vi "Measurement.vi"(8 "error in (no error)":errorcluster, 9 "Grandeza":string, 10 "Multiplicador":dbl, 11 "8846A in":refnum<class "8846A.lvclass">) -> (0 "error out":errorcluster, 2 "Measurement":dbl, 3 "8846A out":refnum<class "8846A.lvclass">)   [LabVIEW 2015, in "8846A.lvclass"]
doc: "VI used to measure Value using the multimeter"
uses:
  8846A.lvclass
  <instrlib>/Fluke 884X Series/Public/Data/Read (Single Point).vi
  <instrlib>/Fluke 884X Series/Fluke 884X Series.lvlib
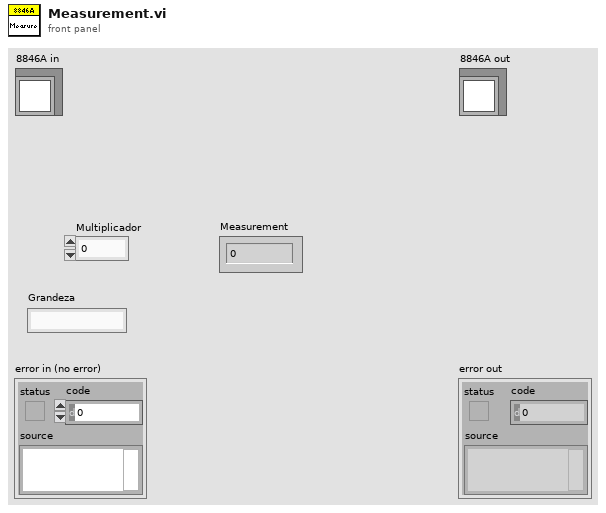
[diagram p1: front panel]
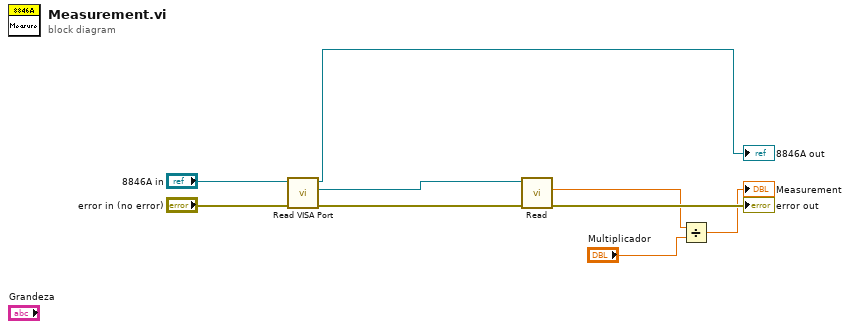
[diagram p0: block diagram]
diagram:
  n1 = call-dynamic "Read VISA Port.vi"("error in (no error)"="error in (no error)", "Device in"="8846A in") -> ("error out"=w4:errorcluster, "VISA Port"=w5:refnum<visa-resource-name>, "Device out"=→"8846A out":refnum<class "8846A.lvclass">)  [unwired: 7 in]
  n2 = call-poly <instrlib>:"Read.vi"("error in (no error)"=w4, "VISA resource name"=w5) -> ("error out"=→"error out":errorcluster, "Measurement"=w2:dbl)  [unwired: 7 in, 1 out]
  n3 = Divide(x=w2, y="Multiplicador") -> (x/y=→"Measurement":dbl)
